vi "Get Target Password.vi"(8 "error in (no error)":errorcluster, 11 "Target ref in":refnum<k24>) -> (0 "error out":errorcluster, 2 "Password":string, 3 "Target ref out":refnum<k24>)   [LabVIEW 2019, in "Telemetry Test Utilities.lvlib"]
uses:
  Telemetry Test Utilities.lvlib
  NationalInstruments.VeriStand.SystemDefinitionAPI
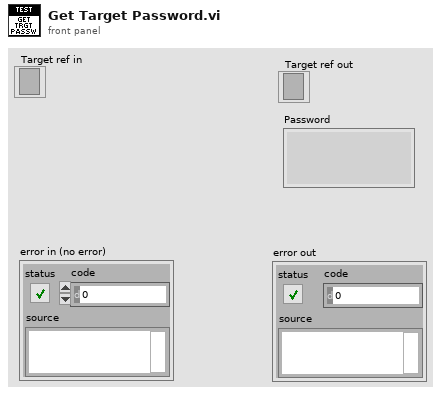
[diagram p1: front panel]
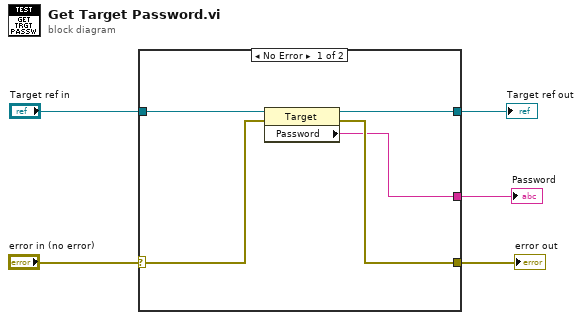
[diagram p0: block diagram]
diagram:
  n1 = case shown="No Error" "error in (no error)" {
    selector: "error in (no error)" -> [w6 w11]
    tunnel: "Target ref in" -> [w10 w12]
    tunnel: [w9 w12] -> w4
    tunnel: [w8 w11] -> w3
    tunnel: [w7 _] -> w2
    frame No Error {
      n2 = property class="Target"(reference=w10, error in=w6) -> (reference out=w9:refnum<k24>, error out=w8:errorcluster, "Password"=w7:string)
    }
    frame Error {
    }
  }
  "Target ref out" <- w4
  "error out" <- w3
  "Password" <- w2
